vi "Save_to_Project.vi"(8 "error in (no error)":errorcluster, 11 "Installer in":refnum<class "Installer.lvclass">) -> (0 "error out":errorcluster, 3 "Installer out":refnum<class "Installer.lvclass">)   [LabVIEW 2020, in "Installer.lvclass"]
uses:
  <vilib>/AppBuilder/IB_Classes/Installer/Installer.lvclass
  <vilib>/AppBuilder/IB_Classes/Installer/Installer.lvclass/Installer.ctl
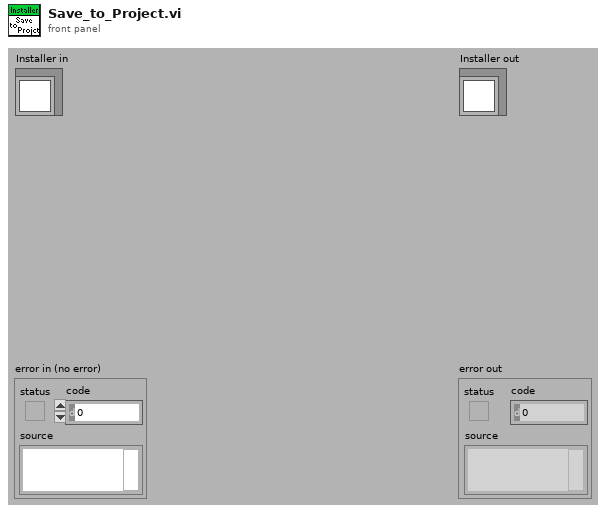
[diagram p1: front panel]
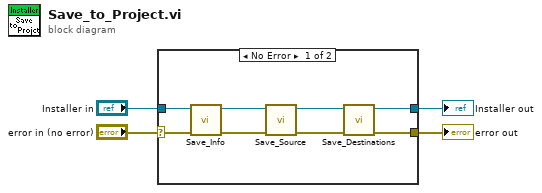
[diagram p0: block diagram]
diagram:
  n1 = case shown="No Error" "error in (no error)" {
    selector: "error in (no error)" -> [w11 w14]
    tunnel: [w5 w14] -> w3
    tunnel: [w7 w13] -> w1
    tunnel: "Installer in" -> [w12 w13]
    frame No Error {
      n2 = call-dynamic "Save_Info.vi"("error in (no error)"=w11, "Class in"=w12) -> ("error out"=w9:errorcluster, "Class out"=w10:refnum<class "Installer.lvclass">)  [unwired: 8 in]
      n3 = call <vilib>:"Save_Source.vi"("error in (no error)"=w9, "Installer in"=w10) -> ("error out"=w6:errorcluster, "Installer out"=w8:refnum<class "Installer.lvclass">)  [unwired: 8 in]
      n4 = call <vilib>:"Save_Destinations.vi"("error in (no error)"=w6, "Installer in"=w8) -> ("error out"=w5:errorcluster, "Installer out"=w7:refnum<class "Installer.lvclass">)  [unwired: 8 in]
    }
    frame Error {
    }
  }
  "error out" <- w3
  "Installer out" <- w1
